vi "PPMS.Command Enum to String.vi"(8 "error in (no error)":errorcluster, 10 "Command":T1, 11 "instrument.PPMS in":refnum<class "instrument.PPMS3.lvclass">) -> (0 "error out":errorcluster, 1 "Commands []":string[](array[string]), 2 "Command":string, 3 "instrument.PPMS out":refnum<class "instrument.PPMS3.lvclass">)   [LabVIEW 2016, in "instrument.PPMS3.lvclass"]
uses:
  instrument.PPMS3.lvclass
  Typedefs/PPMS3.Commands-enum.ctl
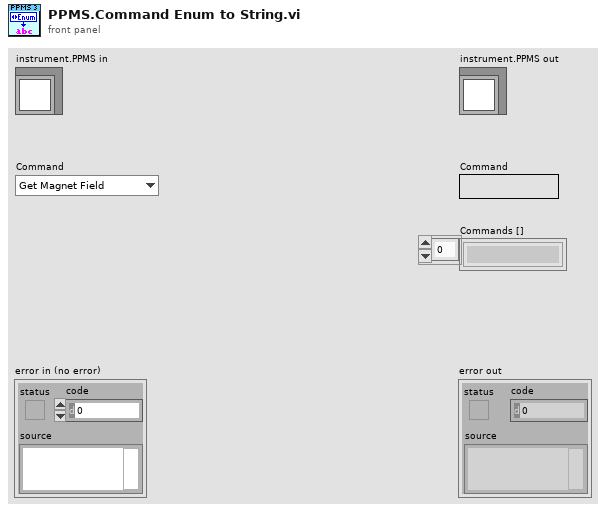
[diagram p1: front panel]
types:
  T1 = typedef "instrument.PPMS3.lvclass/PPMS3.Commands-enum.ctl" = enum16{"Get Magnet Field", "Get Helium Level", "Get Temperature", "Set Magnet Field", "Set Temperature", "getAll"}
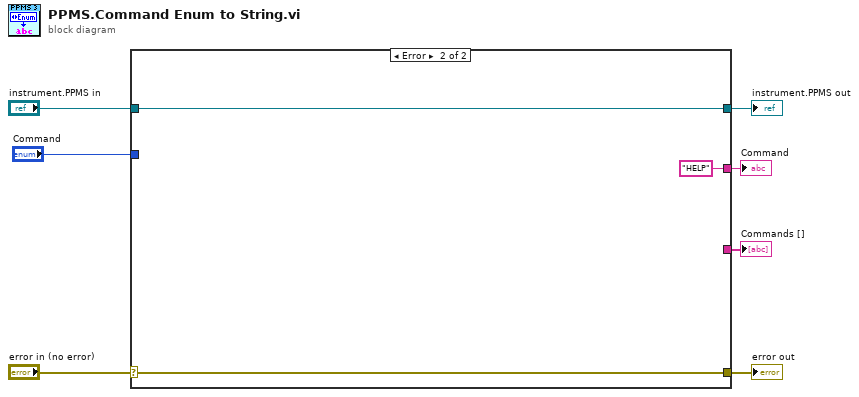
[diagram p0: block diagram]
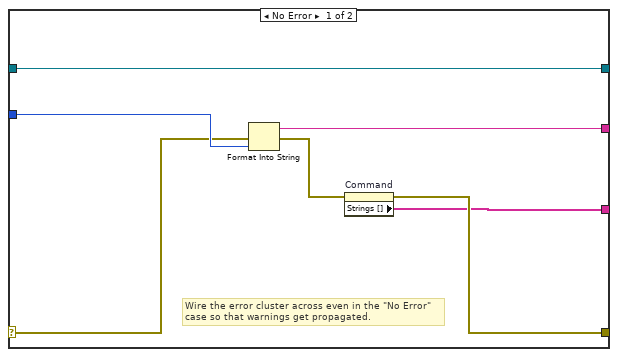
[diagram p2: hidden frame]
diagram:
  n1 = case shown="Error" "error in (no error)" {
    selector: "error in (no error)" -> [w11 w17]
    tunnel: [w10 w17] -> w6
    tunnel: [w14 w16] -> w4
    tunnel: "instrument.PPMS in" -> [w14 w16]
    tunnel: "Command" -> [w12 _]
    tunnel: [w9 "HELP"] -> w1
    tunnel: [w8 _] -> w2
    frame No Error {
      # "Wire the error cluster across even in the \"No Error\"\ncase so that warnings get propagated."
      n2 = Format Into String(error in=w11, w12) -> (resulting string=w9:string, error out=w13:errorcluster)  [unwired: 2 in]
      n3 = property on="Command" class="Enum (strict)"(error in=w13) -> (error out=w10:errorcluster, "Strings []"=w8:string[])  [unwired: 1 in, 1 out]
    }
    frame Error {
    }
  }
  "error out" <- w6
  "instrument.PPMS out" <- w4
  "Commands []" <- w2
  "Command" <- w1
